vi "log header (seq) (SubVI).vi"(10 "字符串":string, 11 "队列输入":refnum<queue>) -> ()   [LabVIEW 2019, in "Take Seq.lvlib"]
uses:
  Take Seq.lvlib
  config.ctl
  Instrument.ctl
  lib/QDInstrument.dll
  <vilib>/NI/Modbus Library/API/Master/Modbus Master.lvclass
  335 state.ctl
panel:
  # "(真是通道1，假是通道2)"
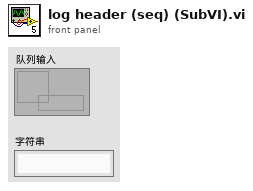
[diagram p1: front panel]
types:
  T1 = enum16{"open", "replace", "create", "open or create", "replace or create", "replace or create with confirmation"}
  T2 = typedef "config.ctl" = cluster{"initialize":string, "6221":cluster{"6221 Resource":refnum<visa-resource-name>, "Delta status":bool}, "7001":cluster{"Ch":bool}, "SR830+6221":cluster{"source":u16, "阻抗":dbl, "量程入 4":i32, "量程入 3":i32, "量程入 2":i32, "量程入 1":i32, "电流":dbl, "SR830 2":bool, "SR830 3":bool, "SR830 4":bool, "SR830 1":bool, "VISA 1":refnum<visa-resource-name>, "VISA 2":refnum<visa-resource-name>, "VISA 3":refnum<visa-resource-name>, "VISA 4":refnum<visa-resource-name>, "量程":enum16{"量程每次测量会判定", "量程不变为设定值"}}, "2400":cluster{"2400":bool, "VISA":refnum<visa-resource-name>}, "ch":cluster{"ch str":string, "ch1":bool, "ch2":bool, "布尔":bool}, "error":bool, "数据文件路径":path, "log":cluster{"log路径":path, "log interval":dbl}, "Instrument":T3}
  T3 = typedef "Instrument.ctl" = cluster{"335 Resource":refnum<visa-resource-name>, "Input (0:A)":u16, "Instrument Type":i32, "quantum design":refnum<k24>, "Heater Output (1:1)":u16, "semaphore":T4, "TCP master instance":refnum<class "Modbus Master.lvclass">, "335 Status":refnum<vi>, "M24C Resource":refnum<visa-resource-name>, "4G supply":refnum<visa-resource-name>, "Temp Status 24C":refnum<vi>, "4g supply status":refnum<vi>}
  T4 = typedef "Semaphore RefNum" = refnum<k1>
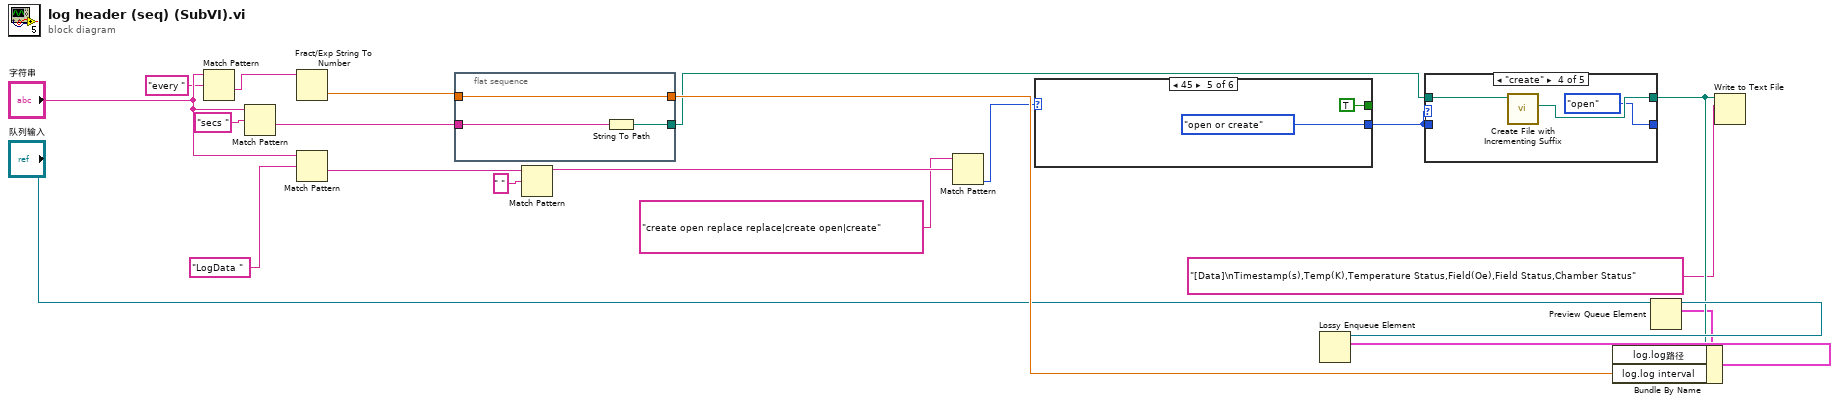
[diagram p0: block diagram]
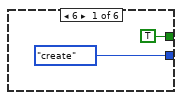
[diagram p6: hidden frame]
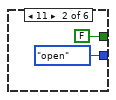
[diagram p7: hidden frame]
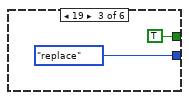
[diagram p8: hidden frame]
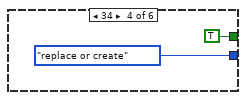
[diagram p9: hidden frame]
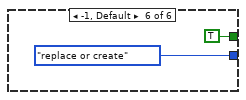
[diagram p10: hidden frame]
diagram:
  n1 = Match Pattern(string="字符串", regular expression="every " ("正则表达式")) -> (after substring=w7:string)  [unwired: 1 in, 3 out]
  n2 = Match Pattern(string="字符串", regular expression="secs " ("正则表达式")) -> (after substring=w9:string)  [unwired: 1 in, 3 out]
  n3 = Fract/Exp String To Number(string=w7) -> (number=w14:dbl)  [unwired: 3 in, 1 out]
  n4 = Match Pattern(string="字符串", regular expression="LogData " ("正则表达式")) -> (after substring=w12:string)  [unwired: 1 in, 3 out]
  n5 = flat-sequence {
    tunnel: [w24] -> w4
    tunnel: w9 -> [w23]
    tunnel: w14 -> [w22]
    tunnel: [w22] -> w19
    frame #0 {
      n6 = String To Path(string=w23) -> (path=w24:path)
    }
  }
  n7 = Match Pattern(string=w12, regular expression=" " ("正则表达式")) -> (before substring=w13:string)  [unwired: 1 in, 3 out]
  n8 = Match Pattern(string="create open replace replace|create open|create" ("字符串"), regular expression=w13) -> (offset past match=w3:i32)  [unwired: 1 in, 3 out]
  n9 = case shown="45" w3 {
    tunnel: [T1."create" ("操作(0:open)") T1."open" ("操作(0:open)") T1."replace" ("操作(0:open)") T1."replace or create" ("操作(0:open)") T1."open or create" ("操作(0:open)") T1."replace or create" ("操作(0:open)")] -> w5
    tunnel: [TRUE FALSE TRUE TRUE TRUE TRUE] -> _
    frame 6 {
    }
    frame 11 {
    }
    frame 19 {
    }
    frame 34 {
    }
    frame 45 {
    }
    frame -1, Default {
    }
  }
  n10 = case shown="\"create\"" w5 {
    tunnel: w4 -> [w38 w40 w42 w45 w47]
    tunnel: [w38 w40 w42 w44 w47] -> w18
    tunnel: [w37 w39 w41 T1."open" ("操作(0:open)") w46] -> _
    tunnel: w5 -> [w37 w39 w41 _ w46]
    frame "open", Default {
    }
    frame "replace" {
    }
    frame "replace or create" {
    }
    frame "create" {
      n11 = call <vilib>:"Create File with Incrementing Suffix.vi"("file path"=w45) -> ("actual path"=w44:path)  [unwired: 8 in, 2 out]
    }
    frame "open or create" {
    }
  }
  n12 = Preview Queue Element(queue="队列输入") -> (queue out=w20:refnum<queue>, element=w17:T2)  [unwired: 2 in, 2 out]
  n13 = Bundle By Name(cluster=w17, "log.log路径"=w18, "log.log interval"=w19) -> (w21:T2)
  n14 = Lossy Enqueue Element(queue=w20, element=w21) -> ()  [unwired: 1 in, 4 out]
  n15 = Write to Text File(file (use dialog)=w18, text="[Data]\nTimestamp(s),Temp(K),Temperature Status,Field(Oe),Field Status,Chamber Status" ("文本")) -> ()  [unwired: 2 in, 3 out]
